vi "AlternatingLEDs.vi"() -> ()   [LabVIEW 2014]
doc: "Ch 4 Do-it-Yourself\n\nThis VI blinks alteratingly 2 LEDs, on PORT 0.0 & 0.1 ."
panel:
  in  "stop":bool
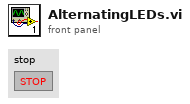
[diagram p1: front panel]
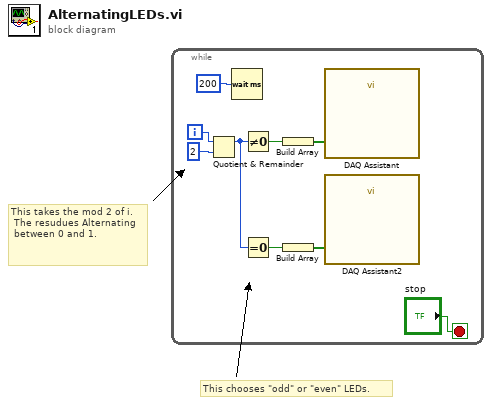
[diagram p0: block diagram]
diagram:
  # "This chooses \"odd\" or \"even\" LEDs."
  # "This takes the mod 2 of i.\n The resudues Alternating\n between 0 and 1."
  n1 = while {
    i -> [w7]
    stop <- "stop" stop-if-true
    n2 = Quotient & Remainder(x=w7, y=2) -> (x-y*floor(x/y)=w4:i32)  [unwired: 1 out]
    n3 = Wait (ms)(milliseconds to wait=u32 200) -> ()  [unwired: 1 out]
    n4 = Not Equal To 0?(x=w4) -> (x != 0?=w3:bool)
    n5 = Equal To 0?(x=w4) -> (x = 0?=w5:bool)
    n6 = Build Array(w3) -> (w1:bool[])
    n7 = Build Array(w5) -> (w2:bool[])
    n8 = call "DAQ Assistant"("data"=w1) -> ()  [unwired: 17 in, 2 out]
    n9 = call "DAQ Assistant2"("data"=w2) -> ()  [unwired: 17 in, 2 out]
  }
